vi "ADQ214 SPI Send.vi"(0 "adq_cu_ptr":u32, 1 "length":u8, 2 "ret":u32, 5 "adq214_num":i32, 7 "addr":u8, 9 "data":string, 11 "error in (no error)":errorcluster, 12 "negedge":bool) -> (4 "adq_cu_ptr out":u32, 6 "ret out":u32, 8 "function return":u32, 15 "error out":errorcluster)   [LabVIEW 8.6, in "ADQAPI.lvlib"]
doc: "extern \"C\" __declspec(dllimport) unsigned int ADQ214_SPISend(void* adq_cu_ptr, int adq214_num, unsigned char addr, const char* data, unsigned char length, bool negedge, unsigned int* ret);"
uses:
  ADQAPI.lvlib
  F:/HRT/Sp Devices Thesis/ADQ-214 project (H R)/ADQAPI.dll
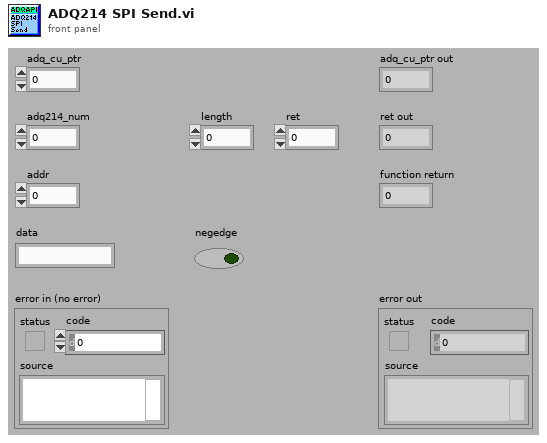
[diagram p1: front panel]
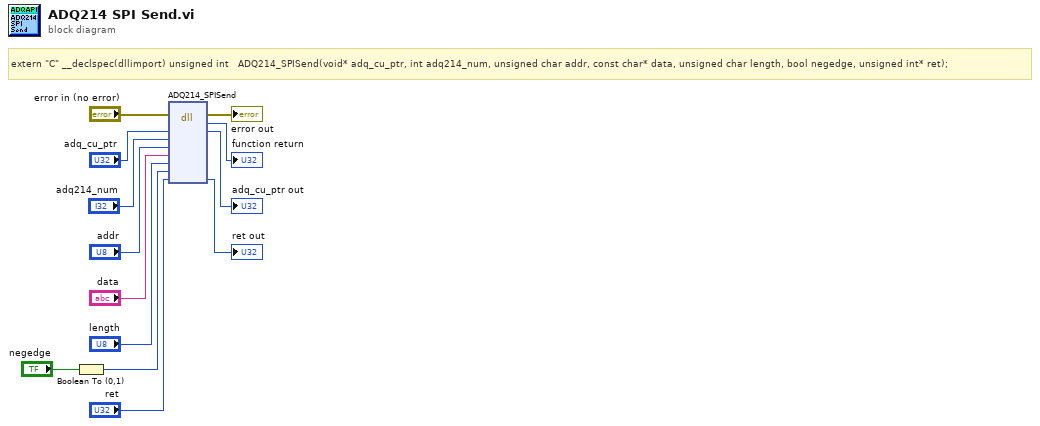
[diagram p0: block diagram]
diagram:
  # "extern \"C\" __declspec(dllimport) unsigned int   ADQ214_SPISend(void* adq_cu_ptr, int adq214_num, unsigned char addr, const char* data, unsigned char length, bool negedge, unsigned int* ret);"
  n1 = Boolean To (0,1)(Boolean="negedge") -> (0, 1=w5:i16)
  n2 = dll-call lib="F:/HRT/Sp Devices Thesis/ADQ-214 project (H R)/ADQAPI.*" fn="ADQ214_SPISend"(error in="error in (no error)", "adq_cu_ptr"="adq_cu_ptr", "adq214_num"="adq214_num", "addr"="addr", "data"="data", "length"="length", "negedge"=w5, "ret"="ret") -> (error out=→"error out":errorcluster, →"function return":u32, "adq_cu_ptr"=→"adq_cu_ptr out":u32, "ret"=→"ret out":u32)  [unwired: 7 in, 1 out]
